vi "pl1000GetValues.vi"(0 "pl1000 handle":i16, 5 "noOfValues":u32, 7 "nOfChannels":u32, 11 "error in (no error)":errorcluster) -> (4 "pl1000 handle out":i16, 6 "values":u16[](array[numeric]), 8 "overflow":bool[](array[boolean]), 10 "noOfValues collected":u32, 14 "triggerIndex":u32, 15 "error out":errorcluster)   [LabVIEW 2016, in "pl1000.lvlib"]
doc: "This function is used to get values after calling pl1000Run \n\nvalues: an array of sample values returned by the function. The size of this buffer must be the number of enabled channels multiplied by the number of samples to be collected.\n\nnoOfValues: the number of sample values per channel that the function should collect. \n\nnOfChannels: the number of channels the device is configured to read data from.\n\noverflow: a bit field indicating which, if any, input channels overflowed the input range of the device. A bit set to 1 indicates an overflow. The least significant bit corresponds to channel 1. May be NULL if an overflow warning is not required. \n\nnoOfValues collecetd: the number of samples per channel that were actually written to the buffer. \n\ntriggerIndex: a number indicating when the trigger event occurred. The number is a zero-based index to the values array, or 0xFFFFFFFF if the information is not available."
uses:
  pl1000.lvlib
  pl1000.dll
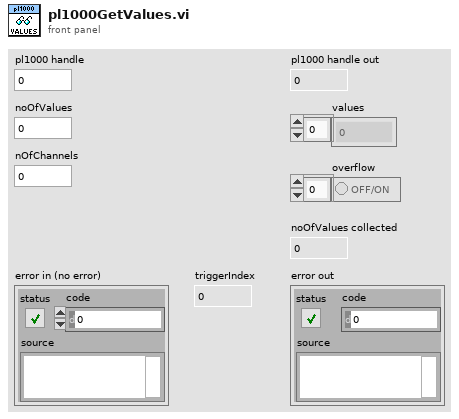
[diagram p1: front panel]
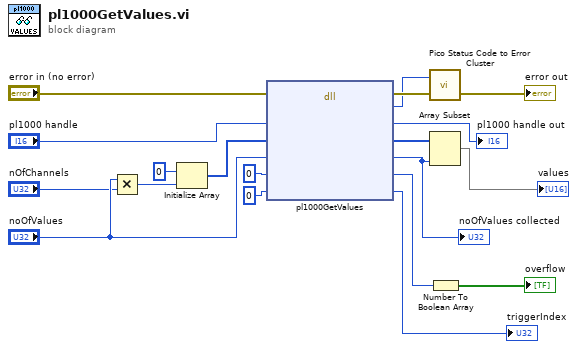
[diagram p0: block diagram]
diagram:
  n1 = Multiply(x="noOfValues", y="nOfChannels") -> (x*y=w4:u32)
  n2 = Initialize Array(u16 0, w4) -> (w3:u16[])
  n3 = dll-call lib="pl1000.dll" fn="pl1000GetValues"(error in="error in (no error)", "handle"="pl1000 handle", "values"=w3, "noOfValues"="noOfValues", "overflow"=u16 0, "triggerIndex"=u32 0) -> (error out=w17:errorcluster, "status"=w16:u32, "handle"=→"pl1000 handle out":i16, "values"=w13:u16[], "noOfValues"=w1:u32, "overflow"=w12:u16, "triggerIndex"=→"triggerIndex":u32)  [unwired: 2 in, 1 out]
  "noOfValues collected" <- w1
  n4 = call "Pico Status Code to Error Cluster.vi"("error in"=w17, "PICO_STATUS"=w16) -> ("error out"=→"error out":errorcluster)  [unwired: 1 in]
  n5 = Array Subset(array=w13, length=w1) -> (→"values":u16[])  [unwired: 1 in]
  n6 = Number To Boolean Array(number=w12) -> (Boolean array=→"overflow":bool[])
